vi "Q_Get Total Distance in KM by type.vi"(8 "error in (no error)":errorcluster, 11 "Data Manager in":refnum<class "Data Manager.lvclass">) -> (0 "error out":errorcluster, 1 "B Ride":dbl, 2 "A Walk":dbl, 3 "Data Manager out":refnum<class "Data Manager.lvclass">, 4 "Run":dbl, 5 "A Run":dbl, 6 "Walk":dbl, 7 "A Ride":dbl)   [LabVIEW 2020, in "Data Manager.lvclass"]
uses:
  Data Manager.lvclass
  Data Manager.lvclass/Data Manager.ctl
  <vilib>/drjdpowell/SQLite Library/SQL Connection/Execute SQL (DBL results).vi
  <vilib>/drjdpowell/SQLite Library/SQLite.lvlib
  <vilib>/drjdpowell/SQLite Library/SQL Connection/Connection.lvclass
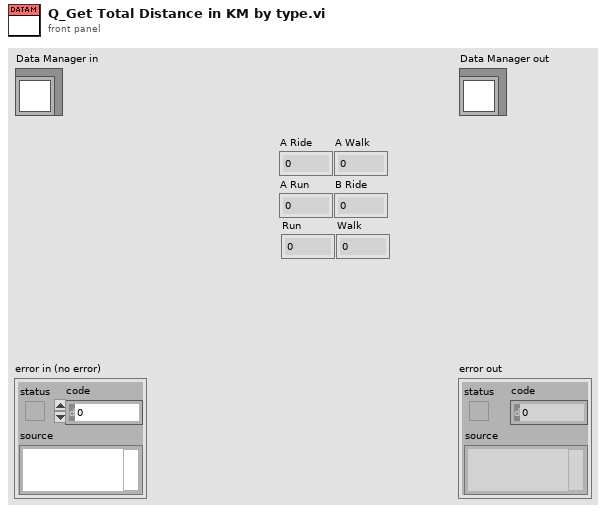
[diagram p1: front panel]
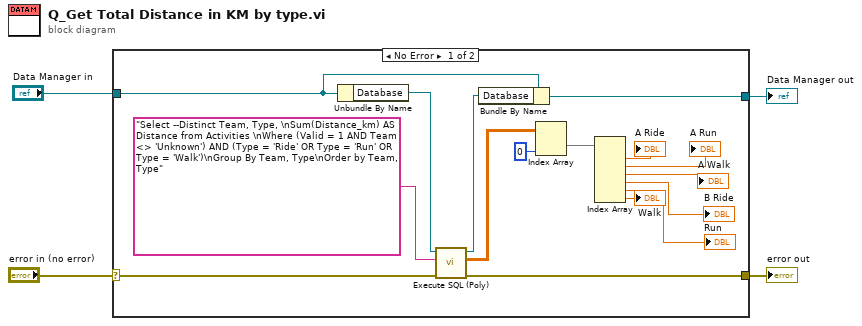
[diagram p0: block diagram]
diagram:
  n1 = case shown="No Error" "error in (no error)" {
    selector: "error in (no error)" -> [w16 w22]
    tunnel: [w15 w22] -> w3
    tunnel: [w18 w21] -> w1
    tunnel: "Data Manager in" -> [w19 w21]
    frame No Error {
      n2 = Unbundle By Name(w19) -> ("Database"=w20:refnum<class "Connection.lvclass">)
      n3 = call-poly <vilib>:"Execute SQL (Poly).vi"("error in (no error)"=w16, "SQL"="Select --Distinct Team, Type, \nSum(Distance_km) AS Distance from Activities \nWhere (Valid = 1 AND Team <> 'Unknown') AND (Type = 'Ride' OR Type = 'Run' OR Type = 'Walk')\nGroup By Team, Type\nOrder by Team, Type", "SQLite Connection in"=w20) -> ("error out"=w15:errorcluster, "Result Set"=w13:dbl[][], "SQLite Connection"=w17:refnum<class "Connection.lvclass">)  [unwired: 5 in, 1 out]
      n4 = Bundle By Name(cluster=w19, "Database"=w17) -> (w18:refnum<class "Data Manager.lvclass">)
      n5 = Index Array(array=w13, index (col)=0 ("disabled index (col)")) -> (element=w11:dbl[])  [unwired: 1 in]
      n6 = Index Array(array=w11) -> (element #1=→"A Ride":dbl, element #2=→"A Run":dbl, element #3=→"A Walk":dbl, element #4=→"B Ride":dbl, element #5=→"Run":dbl, element #6=→"Walk":dbl)  [unwired: 6 in]
    }
    frame Error {
    }
  }
  "error out" <- w3
  "Data Manager out" <- w1
